vi "Read Input B.vi"(8 "error in (no error)":errorcluster, 11 "Subtract_Time in":refnum<class "Subtract_Time-Time.lvclass">) -> (0 "error out":errorcluster, 2 "Abs_Time.lvclass":refnum<class "Abs_Time.lvclass">, 3 "Subtract_Time out":refnum<class "Subtract_Time-Time.lvclass">)   [LabVIEW 2021, in "Subtract_Time-Time.lvclass"]
uses:
  Subtract_Time-Time.lvclass
  Abs_Types/Time/Abs_Time.lvclass
  Subtract_Time-Time.lvclass/Subtract_Time-Time.ctl
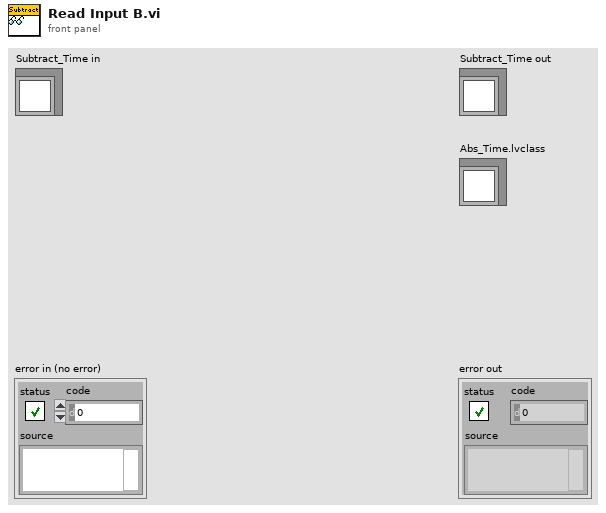
[diagram p1: front panel]
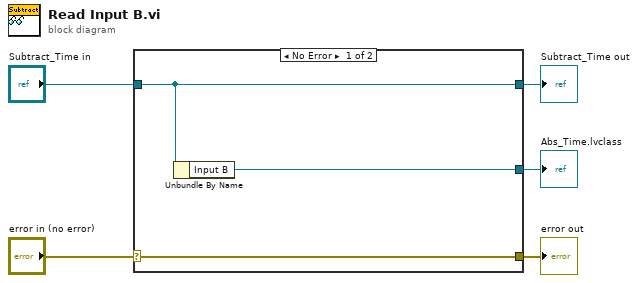
[diagram p0: block diagram]
diagram:
  n1 = case shown="No Error" "error in (no error)" {
    selector: "error in (no error)" -> [w8 w9]
    tunnel: [w8 w9] -> w4
    tunnel: [w7 w10] -> w2
    tunnel: "Subtract_Time in" -> [w7 w10]
    tunnel: [w6 _] -> w1
    frame No Error {
      n2 = Unbundle By Name(w7) -> ("Input B"=w6:refnum<class "Abs_Time.lvclass">)
    }
    frame Error {
    }
  }
  "error out" <- w4
  "Subtract_Time out" <- w2
  "Abs_Time.lvclass" <- w1
